vi "createNewArrayObject.vi"(8 "error in (no error)":errorcluster, 10 "arrayRef":refnum<vi>, 11 "Long in":refnum<class "Long.lvclass">) -> (0 "error out":errorcluster, 3 "Long out":refnum<class "Long.lvclass">)   [LabVIEW 2016, in "Long.lvclass"]
uses:
  Long.lvclass
  D:/Code/ts_SALLabVIEW/SALTypeGenerator/Elements/Numeric/Numeric.lvclass
  <vilib>/numeric/LVNumericRepresentation.ctl
  Numeric/Numeric.lvclass/Numeric.ctl
  Signed/Signed.lvclass
  Numeric/Numeric.lvclass
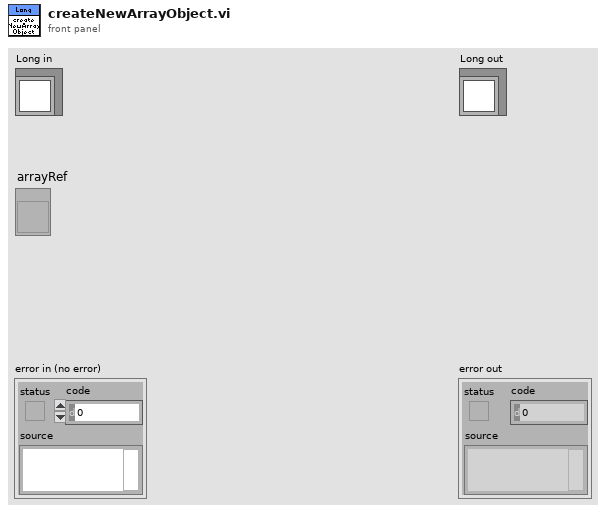
[diagram p1: front panel]
types:
  T1 = typedef "LVNumericRepresentation.ctl" = enum32{"Extended Precision", "Double Precision", "Single Precision", "Long", "Word", "Byte", "Unsigned Long", "Unsigned Word", "Unsigned Byte", "Complex Extended", "Complex Double", "Complex Single", "Quad", "Unsigned Quad", "Fixed-Point"}
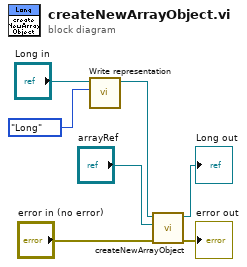
[diagram p0: block diagram]
diagram:
  n1 = call "Write representation.vi"("Numeric Representation"=LVNumericRepresentation."Long", "Numeric in"="Long in") -> ("Numeric out"=w2:refnum<class "Long.lvclass">)  [unwired: 9 in]
  n2 = call-parent "createNewArrayObject.vi"("error in (no error)"="error in (no error)", "arrayRef"="arrayRef", "Numeric in"=w2) -> ("error out"=→"error out":errorcluster, "Numeric out"=→"Long out":refnum<class "Long.lvclass">)  [unwired: 7 in]
